vi "HTTP-GET.vi"(11 "Command":string="GET home.asp HTTP/1.1\nHost: 192.168.16.1\n\n") -> (3 "String":string)   [LabVIEW 2015]
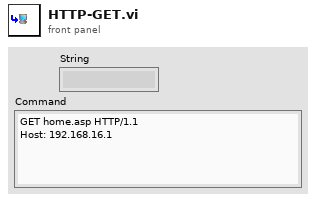
[diagram p1: front panel]
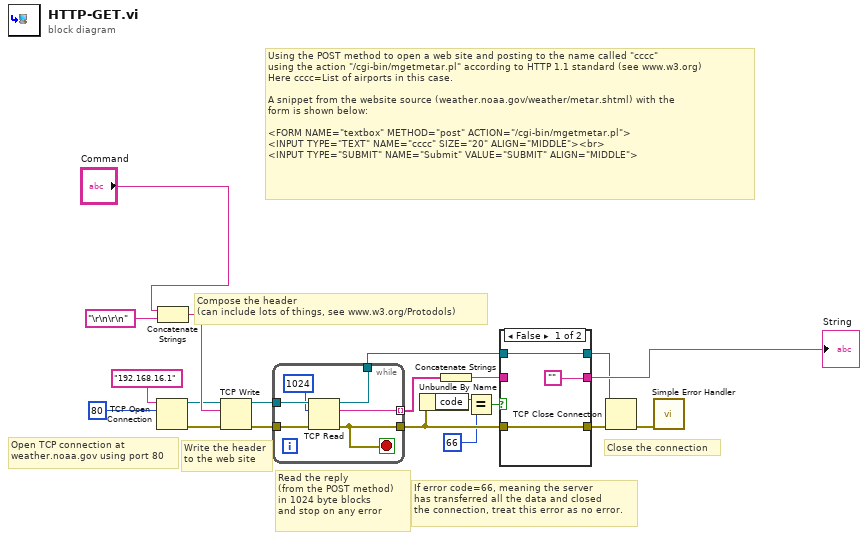
[diagram p0: block diagram]
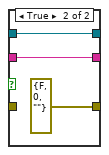
[diagram p2: hidden frame]
diagram:
  # "Compose the header\n(can include lots of things, see www.w3.org/Protodols)"
  # "Close the connection"
  # "If error code=66, meaning the server\nhas transferred all the data and closed\nthe connection, treat this error as no error."
  # "Read the reply\n(from the POST method)\nin 1024 byte blocks\nand stop on any error"
  # "Write the header\nto the web site"
  # "Open TCP connection at\nweather.noaa.gov using port 80"
  # "Using the POST method to open a web site and posting to the name called \"cccc\"\nusing the action \"/cgi-bin/mgetmetar.pl\" according to HTTP 1.1 standard (see www.w3.org)\nHere cccc=List of airports in this case.\n\nA snippet from the website source (weather.noaa.gov/weather/metar.shtml) with the\nform is shown below:\n\n<FORM NAME=\"textbox\" METHOD=\"post\" ACTION=\"/cgi-bin/mgetmetar.pl\">\n<INPUT TYPE=\"TEXT\" NAME=\"cccc\" SIZE=\"20\" ALIGN=\"MIDDLE\"><br>\n<INPUT TYPE=\"SUBMIT\" NAME=\"Submit\" VALUE=\"SUBMIT\" ALIGN=\"MIDDLE\">"
  n1 = TCP Open Connection(address="192.168.16.1", remote port or service name=u16 80 ("remote port")) -> (connection ID=w4:refnum<k5>, error out=w3:errorcluster)  [unwired: 3 in]
  n2 = Concatenate Strings("Command", "\r\n\r\n" ("string")) -> (w5:string)
  n3 = TCP Write(connection ID=w4, data in=w5, error in (no error)=w3) -> (connection ID out=w8:refnum<k5>, error out=w9:errorcluster)  [unwired: 1 in, 1 out]
  n4 = while {
    tunnel: w9 -> [w26]
    tunnel: w8 -> [w25]
    tunnel: [w21] -> w11
    tunnel: [w24] -> w14
    tunnel: [w23] -> w12 mode=indexing
    stop <- w21 stop-if-true
    n5 = TCP Read(connection ID=w25, bytes to read=1024, error in (no error)=w26) -> (connection ID out=w24:refnum<k5>, data out=w23:string, error out=w21:errorcluster)  [unwired: 2 in]
  }
  n6 = Unbundle By Name(w11) -> ("code"=w6:i32)
  n7 = Concatenate Strings(w12) -> (w13:string)
  n8 = Equal?(x=w6, y=66) -> (x = y?=w7:bool)
  n9 = case shown="False" w7 {
    tunnel: ["" w31] -> w19
    tunnel: w13 -> [_ w31]
    tunnel: [w28 errorcluster {"status"=FALSE, "code"=0, "source"=""} ("error in (no error)")] -> w16
    tunnel: w11 -> [w28 _]
    tunnel: w14 -> [w27 w30]
    tunnel: [w27 w30] -> w15
    frame False {
    }
    frame True {
    }
  }
  "String" <- w19
  n10 = TCP Close Connection(connection ID=w15, error in (no error)=w16) -> (error out=w1:errorcluster)  [unwired: 1 in, 1 out]
  n11 = call <vilib>:"Simple Error Handler.vi"("error in (no error)"=w1) -> ()  [unwired: 4 in, 5 out]
